vi "Do.vi"(8 "error in (no error)":errorcluster, 10 "Actor in":refnum<class "Actor.lvclass">, 11 "Update Elevator State Msg":refnum<class "Update Elevator State Msg.lvclass">) -> (0 "error out":errorcluster, 2 "Actor out":refnum<class "Actor.lvclass">)   [LabVIEW 2014, in "Elevator.lvlib" / "Update Elevator State Msg.lvclass"]
doc: "This VI delivers the message to the actor by calling the appropriate method(s) on the actor."
uses:
  Update Elevator State Msg.lvclass
  <vilib>/ActorFramework/Actor/Actor.lvclass
  Elevator State Receiver Class/Elevator State Receiver.lvclass
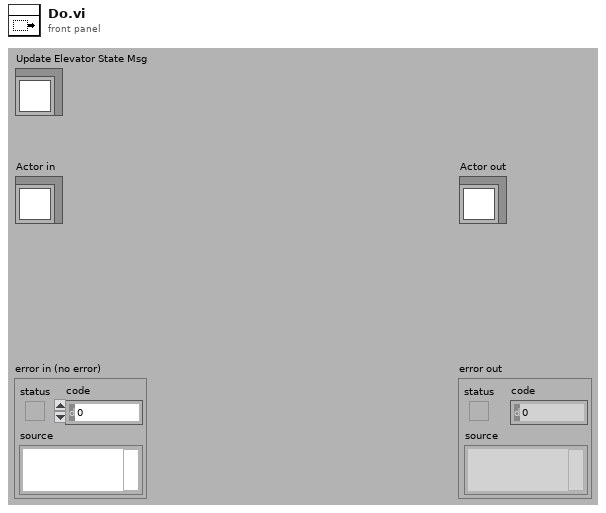
[diagram p1: front panel]
types:
  T1 = typedef "Elevator.lvlib/Elevator.lvclass/Elevator State.ctl" = cluster{"At Bottom":bool, "At Top":bool, "At Setpoint":bool, "Target Rate (RPM)":dbl, "Current Travel Rate":dbl, "Current Elevation":dbl, "Brake On":bool, "Motor Elevate Rate (RPM))":dbl, "Has Been Home":bool}
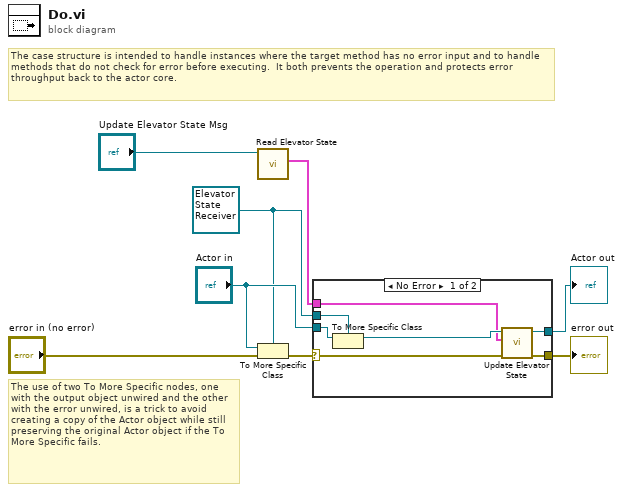
[diagram p0: block diagram]
diagram:
  w3 = refnum<class "Elevator State Receiver.lvclass"> refnum ("Actor in")
  # "The use of two To More Specific nodes, one with the output object unwired and the other with the error unwired, is a trick to avoid creating a copy of the Actor object while still preserving the original Actor object if the To More Specific fails."
  # "The case structure is intended to handle instances where the target method has no error input and to handle methods that do not check for error before executing.  It both prevents the operation and protects error throughput back to the actor core."
  n1 = call-dynamic "Read Elevator State.vi"("Current State Msg in"="Update Elevator State Msg") -> ("Elevator State"=w1:T1)  [unwired: 8 in, 2 out]
  n2 = To More Specific Class(target class=w3, reference="Actor in", error in="error in (no error)") -> (error out=w7:errorcluster)  [unwired: 1 out]
  n3 = case shown="No Error" w7 {
    selector: w7 -> [w13 w17]
    tunnel: [w15 w17] -> w6
    tunnel: [w14 w16] -> w5
    tunnel: "Actor in" -> [w12 w16]
    tunnel: w3 -> [w11 _]
    tunnel: w1 -> [w9 _]
    frame No Error {
      n4 = To More Specific Class(target class=w11, reference=w12) -> (specific class reference=w10:refnum<class "Elevator State Receiver.lvclass">)  [unwired: 1 in, 1 out]
      n5 = call-dynamic "Update Elevator State.vi"("error in (no error)"=w13, "Elevator State"=w9, "Elevator State Receiver in"=w10) -> ("error out"=w15:errorcluster, "Elevator State Receiver out"=w14:refnum<class "Elevator State Receiver.lvclass">)  [unwired: 7 in]
    }
    frame Error {
      # "If type check fails, pass the original object out again."
    }
  }
  "error out" <- w6
  "Actor out" <- w5
